vi "testKeithley.vi"() -> ()   [LabVIEW 2009, in "run.lvlib"]
uses:
  testing/run.lvlib
  K2602.lvclass
panel:
  out "script":string
  in  "physical channels":string="K2606_Ao_00, K2606_Ao_01"
  in  "stop":bool
  in  "data":dbl[][][](array[numeric])
  in  "ConfigArray":T1(array[cluster])=[{"Range"={"current"=3.0, "voltage"=40.0}, "triggering_inUse"={"start_trigger"="K2606_Digio_01", "clock"=""}, "Limits"={"VoltageLimit"=10.0, "CurrentLimit"=1.0}}, {"Range"={"current"=2.0, "voltage"=12.0}, "triggering_inUse"={"start_trigger"="internal", "clock"=""}, "Limits"={"VoltageLimit"=0.5, "CurrentLimit"=3.0}}]
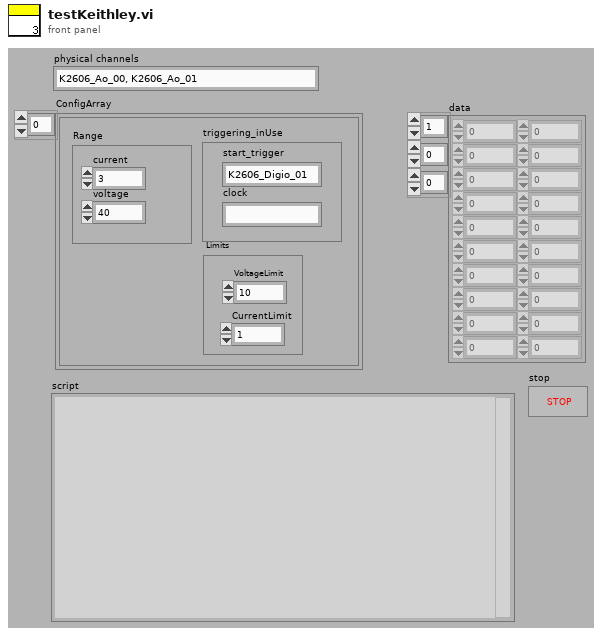
[diagram p1: front panel]
types:
  T1 = cluster{"Range":cluster{"current":dbl, "voltage":dbl}, "triggering_inUse":cluster{"start_trigger":string, "clock":string}, "Limits":cluster{"VoltageLimit":dbl, "CurrentLimit":dbl}}[]
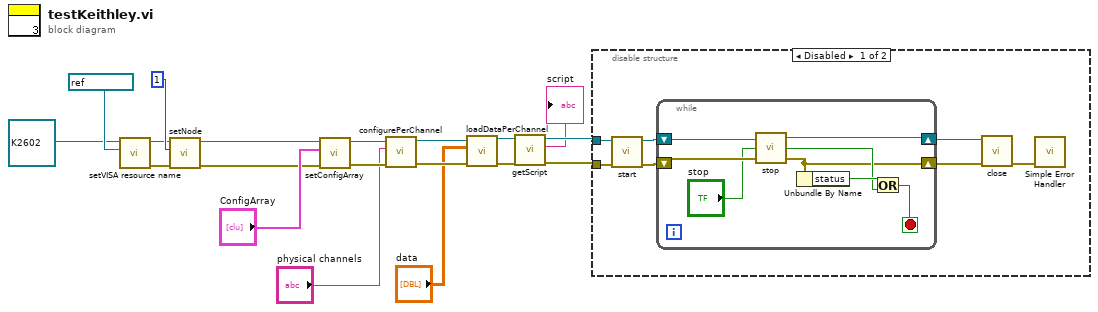
[diagram p0: block diagram]
diagram:
  n1 = call "setVISA resource name.vi"("VISA resource name"=refnum<visa-resource-name> "keithley", "K2602 in"=refnum<class "K2602.lvclass"> refnum ("Hardware:Channels.lvlib:K2602.lvclass")) -> ("error out"=w11:errorcluster, "K2602 out"=w9:refnum<class "K2602.lvclass">)  [unwired: 8 in]
  n2 = call "setNode.vi"("error in (no error)"=w11, "node"=1, "K2602 in"=w9) -> ("error out"=w7:errorcluster, "K2602 out"=w8:refnum<class "K2602.lvclass">)  [unwired: 7 in]
  n3 = call-dynamic "setConfigArray.vi"("error in (no error)"=w7, "ConfigArray"="ConfigArray", "K2602 in"=w8) -> ("error out"=w17:errorcluster, "K2602 out"=w18:refnum<class "K2602.lvclass">)  [unwired: 7 in]
  n4 = call-dynamic "configurePerChannel.vi"("error in (no error)"=w17, "physical channels"="physical channels", "K2602 in"=w18) -> ("error out"=w14:errorcluster, "K2602 out"=w15:refnum<class "K2602.lvclass">)  [unwired: 7 in]
  n5 = call-dynamic "loadDataPerChannel.vi"("error in (no error)"=w14, "data"="data", "K2602 in"=w15) -> ("error out"=w5:errorcluster, "K2602 out"=w6:refnum<class "K2602.lvclass">)  [unwired: 7 in]
  n6 = call "getScript.vi"("error in (no error)"=w5, "K2602 in"=w6) -> ("error out"=w3:errorcluster, "script"=→"script":string, "K2602 out"=w4:refnum<class "K2602.lvclass">)  [unwired: 7 in]
  n7 = disable-structure shown="Disabled" {
    disable-tunnel: w4 -> [w26 _]
    disable-tunnel: w3 -> [w25 _]
    frame #0 {
      n8 = call-dynamic "start.vi"("error in (no error)"=w25, "K2602 in"=w26) -> ("error out"=w23:errorcluster, "K2602 out"=w24:refnum<class "K2602.lvclass">)  [unwired: 8 in]
      n9 = while {
        shift-right: [w33] -> w22
        shift-left: w24 -> [w34]
        shift-right: [w27] -> w21
        shift-left: w23 -> [w32]
        stop <- w28 stop-if-true
        n10 = call-dynamic "stop.vi"("error in (no error)"=w32, "stop"="stop", "K2602 in"=w34) -> ("error out"=w27:errorcluster, "Stopped"=w29:bool, "K2602 out"=w33:refnum<class "K2602.lvclass">)
        n11 = Unbundle By Name(w27) -> ("status"=w30:bool)
        n12 = Or(x=w30, y=w29) -> (x .or. y?=w28:bool)
      }
      n13 = call-dynamic "close.vi"("error in (no error)"=w21, "K2602 in"=w22) -> ("error out"=w20:errorcluster)  [unwired: 9 in]
      n14 = call <vilib>:"Simple Error Handler.vi"("error in (no error)"=w20) -> ()  [unwired: 4 in, 5 out]
    }
    frame #1 {
    }
  }
